vi "press_stop.vi"(6 "Attempt stop on error? (T)":bool=TRUE, 7 "Abort VI if necessary?":bool caption="Abort VI if necessary? (F)", 8 "error in":errorcluster, 9 "button names (stop, stop?)":string[](array[string])=["stop", "Stop", "stop?", "Stop?"], 10 "Timeout before close":i32=2000 caption="Timeout before close (2k ms)" min=-1, 11 "vi ref":refnum<vi>) -> (0 "error out":errorcluster, 2 "VI aborted?":bool, 3 "VI path":path)   [LabVIEW 2015]
uses:
  polys/poly_is_running_state.vi
  <vilib>/GPower/Timing/Library/Wait/Wait_ms.vi
  <vilib>/GPower/Timing/Library/Remaining/Remaining_ms.vi
  <vilib>/GPower/Error/Library/IsError.vi
  polys/poly_control_signalling_write_single.vi
  <vilib>/GPower/Timing/GPTiming.lvlib
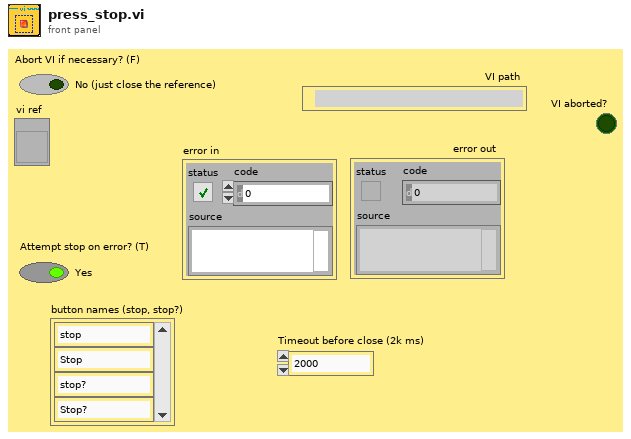
[diagram p1: front panel]
types:
  T1 = enum16{"Val", "Val(Sgnl)", "Val(Undo)", "Method"}
  T2 = enum32{"Bad", "Idle", "Run top level", "Running"}
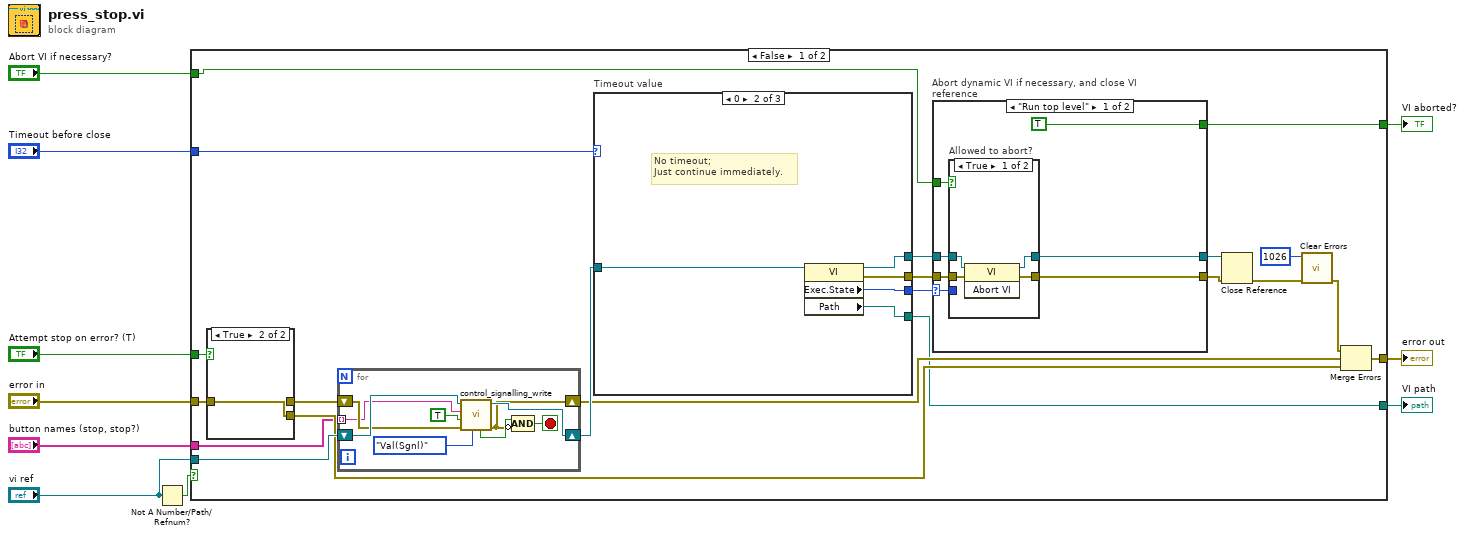
[diagram p0: block diagram]
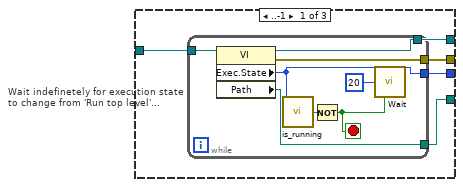
[diagram p2: hidden frame]
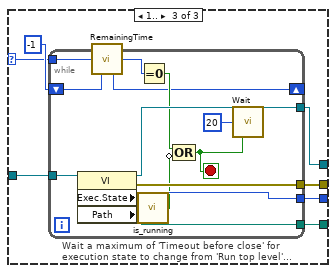
[diagram p3: hidden frame]
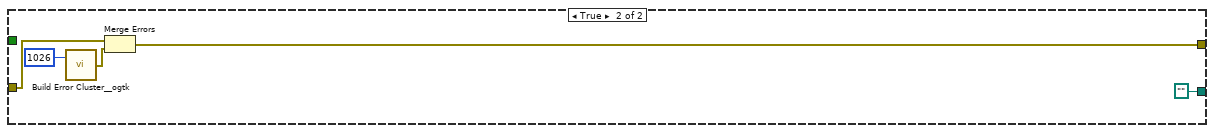
[diagram p7: hidden frame]
diagram:
  n1 = Not A Number/Path/Refnum?(number/path/refnum="vi ref") -> (NaN/Path/Refnum?=w1:bool)
  n2 = case shown="False" w1 {
    tunnel: "vi ref" -> [w31 _]
    tunnel: "Attempt stop on error? (T)" -> [w30 _]
    tunnel: "error in" -> [w29 w99]
    tunnel: [w26 w98] -> w8
    tunnel: "Timeout before close" -> [w25 _]
    tunnel: "Abort VI if necessary?" -> [w21 _]
    tunnel: [w18 _] -> w5
    tunnel: [w17 path ""] -> w4
    tunnel: "button names (stop, stop?)" -> [w11 _]
    frame False {
      n3 = case shown="True" w30 {
        tunnel: [_ w86] -> w27
        tunnel: w29 -> [w85 w86]
        tunnel: [w85 _] -> w28
        frame False {
        }
        frame True {
        }
      }
      n4 = for {
        shift-right: [w93] -> w20
        shift-left: w31 -> [w94]
        tunnel: w11 -> [w89] mode=indexing
        shift-right: [w87] -> w19
        shift-left: w28 -> [w92]
        stop <- w95 stop-if-true
        n5 = call-poly "control_signalling_write.vi"("mode (Sgnl)"=T1."Val(Sgnl)", "error in (no error)"=w92, "Value"=TRUE, "Control Name"=w89, "vi reference"=w94) -> ("error out"=w87:errorcluster, "vi reference out"=w93:refnum<vi>, "found?"=w88:bool)  [unwired: 3 in, 1 out]
        n6 = Compound Arithmetic op=AND(w88, invert w87) -> (w95:bool)
      }
      n7 = case "Timeout value" shown="0" w25 {
        selector: w25 -> [_ _ w50]
        tunnel: w20 -> [w36 w49 w56]
        tunnel: [w35 w48 w55] -> w24
        tunnel: [w34 w47 w54] -> w23
        tunnel: [w33 w46 w53] -> w22
        tunnel: [w32 w45 w52] -> w17
        frame ..-1 {
          n8 = while "Wait indefinetely for execution state\nto change from 'Run top level'..." {
            tunnel: w36 -> [w44]
            tunnel: [w43] -> w35
            tunnel: [w39] -> w34
            tunnel: [w42] -> w33
            tunnel: [w41] -> w32
            stop <- w37 stop-if-true
            n9 = property class="VI"(reference=w44) -> (reference out=w43:refnum<vi>, error out=w42:errorcluster, "Exec.State"=w39:T2, "Path"=w41:path)  [unwired: 1 in]
            n10 = call-poly "is_running.vi"("execution state"=w39) -> ("running top level?"=w38:bool)  [unwired: 4 in]
            n11 = Not(x=w38) -> (.not. x?=w37:bool)
            n12 = call-poly <vilib>:"Wait.vi"("Time to wait"=20 ("milliseconds to wait"), "Skip wait?"=w37) -> ()  [unwired: 13 in, 1 out]
          }
        }
        frame 0 {
          # "No timeout;\nJust continue immediately."
          n13 = property class="VI"(reference=w49) -> (reference out=w48:refnum<vi>, error out=w46:errorcluster, "Exec.State"=w47:T2, "Path"=w45:path)  [unwired: 1 in]
        }
        frame 1.. {
          n14 = while "Wait a maximum of 'Timeout before close' for\nexecution state to change from 'Run top level'..." {
            tunnel: w56 -> [w69]
            tunnel: [w68] -> w55
            tunnel: [w58] -> w54
            tunnel: [w67] -> w53
            tunnel: [w66] -> w52
            shift-right: [w61] -> _
            shift-left: i64 -1 ("Start time out") -> [w62]
            tunnel: w50 -> [w64]
            stop <- w60 stop-if-true
            n15 = property class="VI"(reference=w69) -> (reference out=w68:refnum<vi>, error out=w67:errorcluster, "Exec.State"=w58:T2, "Path"=w66:path)  [unwired: 1 in]
            n16 = call-poly <vilib>:"RemainingTime.vi"("Time period target"=w64, "Start time in"=w62) -> ("Remaining time"=w63:i32, "Start time out"=w61:i64)  [unwired: 9 in, 3 out]
            n17 = call-poly "is_running.vi"("execution state"=w58) -> ("running top level?"=w57:bool)  [unwired: 4 in]
            n18 = Equal To 0?(x=w63) -> (x = 0?=w65:bool)
            n19 = Compound Arithmetic op=OR(w65, invert w57) -> (w60:bool)
            n20 = call-poly <vilib>:"Wait.vi"("Time to wait"=20 ("milliseconds to wait"), "Skip wait?"=w60) -> ()  [unwired: 13 in, 1 out]
          }
        }
      }
      n21 = case "Abort dynamic VI if necessary, and close VI reference" shown="\"Run top level\"" w23 {
        selector: w23 -> [w72 _]
        tunnel: w24 -> [w76 w84]
        tunnel: w22 -> [w75 w83]
        tunnel: [TRUE _] -> w18
        tunnel: w21 -> [w73 _]
        tunnel: [w71 w83] -> w14
        tunnel: [w70 w84] -> w12
        frame "Run top level" {
          n22 = case "Allowed to abort?" shown="True" w73 {
            tunnel: w76 -> [w80 w81]
            tunnel: w75 -> [w79 w82]
            tunnel: [w78 w82] -> w71
            tunnel: w72 -> [_ _]
            tunnel: [w77 w81] -> w70
            frame True {
              n23 = invoke class="VI" method="Abort VI"(reference=w80, error in=w79) -> (reference out=w77:refnum<vi>, error out=w78:errorcluster)  [unwired: 1 in, 1 out]
            }
            frame False {
            }
          }
        }
        frame "Bad", "Idle", "Running" {
        }
      }
      n24 = Close Reference(reference=w12, error in (no error)=w14) -> (error out=w13:errorcluster)
      n25 = call <vilib>:"Clear Errors.vi"("error in (no error)"=w13, "specific error code to clear (0: all)"=1026) -> ("error out"=w16:errorcluster)  [unwired: 4 in, 1 out]
      n26 = Merge Errors(w16, w19, w27) -> (w26:errorcluster)
    }
    frame True {
      n27 = call <userlib>:"Build Error Cluster__ogtk.vi"("code"=1026) -> ("error out"=w97:errorcluster)  [unwired: 1 in]
      n28 = Merge Errors(w99, w97) -> (w98:errorcluster)
    }
  }
  "VI path" <- w4
  "VI aborted?" <- w5
  "error out" <- w8
